vi "Update Joints.vi"(8 "error in (no error)":errorcluster, 9 "Scale (1)":dbl=1.0, 10 "Joints":sgl[](array[numeric]), 11 "Joint Array":T1[](array[typedef])) -> (0 "error out":errorcluster)   [LabVIEW 2017, in "NI_Robotics_3DKinematics.lvlib"]
uses:
  <vilib>/robotics/Kinematics/Plotting/NI_Robotics_3DKinematics.lvlib
  <vilib>/robotics/Kinematics/Plotting/Joint Control.ctl
  <vilib>/robotics/Kinematics/Plotting/Joint Type.ctl
  <vilib>/Analysis/baseanly.llb/Real A x B.vi
  <vilib>/Analysis/_algsub.llb/Vector Norm.vi
  <vilib>/Analysis/_algsub.llb/Real Vector Norm.vi
  <vilib>/Analysis/baseanly.llb/Outer Product.vi
  <vilib>/Analysis/baseanly.llb/Real Outer Product.vi
  <vilib>/robotics/Kinematics/Create Lie Group Matrix.vi
  <vilib>/Utility/AngleManip/Degrees to Radians (Scalar DBL).vi
  <vilib>/Analysis/Matrix/Numeric/Add/Add.vi
  <vilib>/Analysis/Matrix/Numeric/Add/Add - RM,RM.vi
  <vilib>/Analysis/Matrix/Numeric/Multiply/Multiply.vi
  <vilib>/Analysis/Matrix/Numeric/Multiply/Multiply - R,RM.vi
  <vilib>/Analysis/Matrix/Numeric/Multiply/Multiply - RM,R.vi
  <vilib>/Analysis/7linalg.llb/Create Special Matrix.vi
  <vilib>/Analysis/7linalg.llb/Create Special Real Matrix.vi
  <vilib>/picture/3D Picture Control/NI_3D Picture Control.lvlib
  <vilib>/Utility/AngleManip/NI_AngleManipulation.lvlib
  <vilib>/robotics/Kinematics/NI_Kinematics.lvlib
  <vilib>/Analysis/NI_AALBase.lvlib
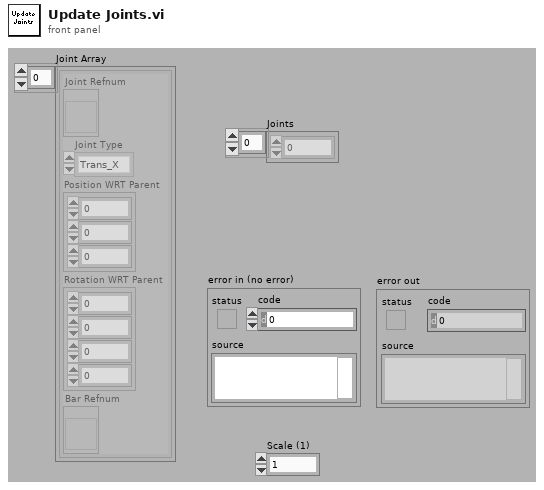
[diagram p1: front panel]
types:
  T1 = typedef "NI_Robotics_3DKinematics.lvlib/Joint Control.ctl" = cluster{"Joint Refnum":refnum<vi>, "Joint Type":T2, "Position WRT Parent":dbl[], "Rotation WRT Parent":dbl[], "Bar Refnum":refnum<vi>}
  T2 = typedef "NI_Robotics_3DKinematics.lvlib/Joint Type.ctl" = enum16{"Trans_X", "Trans_Y", "Trans_Z", "Rot_X", "Rot_Y", "Rot_Z", "None"}
  T3 = cluster{"Position WRT Parent[0]":dbl, "Position WRT Parent[1]":dbl, "Position WRT Parent[2]":dbl}
  T4 = cluster{"Rotation WRT Parent[0]":dbl, "Rotation WRT Parent[1]":dbl, "Rotation WRT Parent[2]":dbl}
  T5 = typedef "NI_Matrix.lvlib/RealMatrix.ctl" = dbl[][]
  T6 = cluster{"A x B[0]":dbl, "A x B[1]":dbl, "A x B[2]":dbl}
  T7 = cluster{"Numeric":dbl, "Numeric":dbl, "Numeric":dbl}
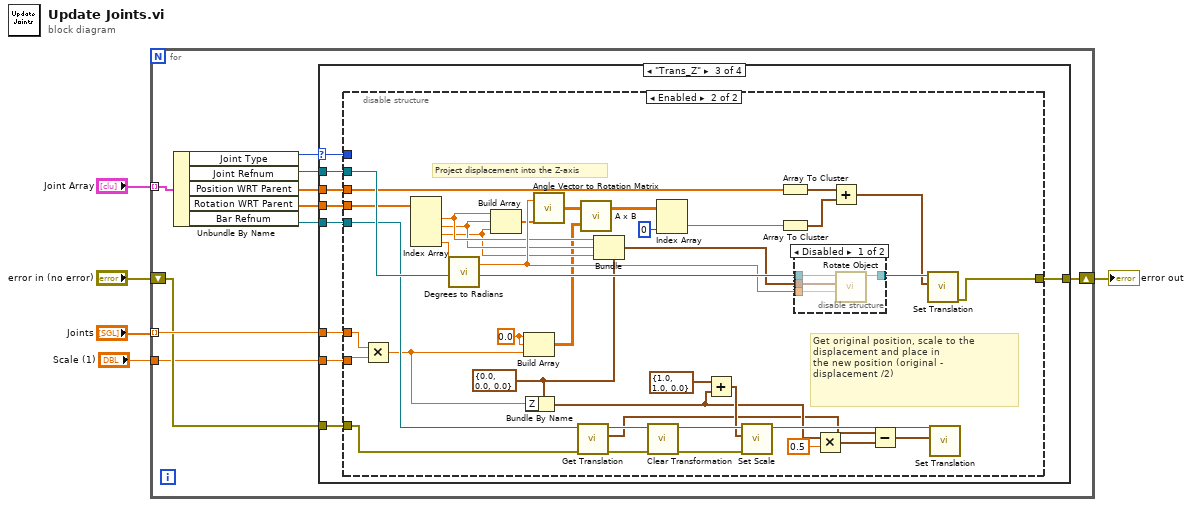
[diagram p0: block diagram]
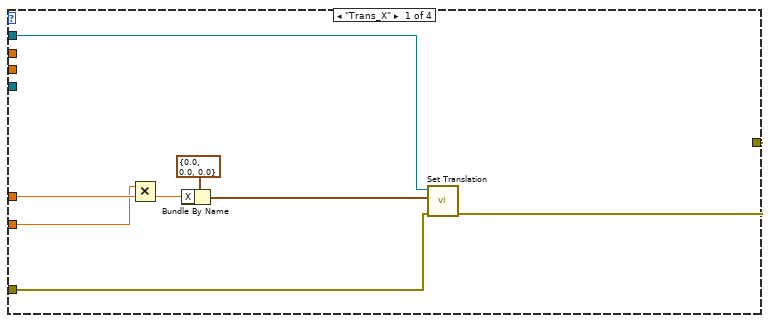
[diagram p2: hidden frame]
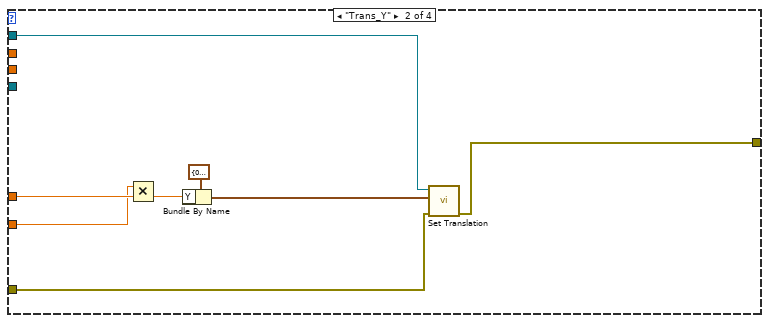
[diagram p3: hidden frame]
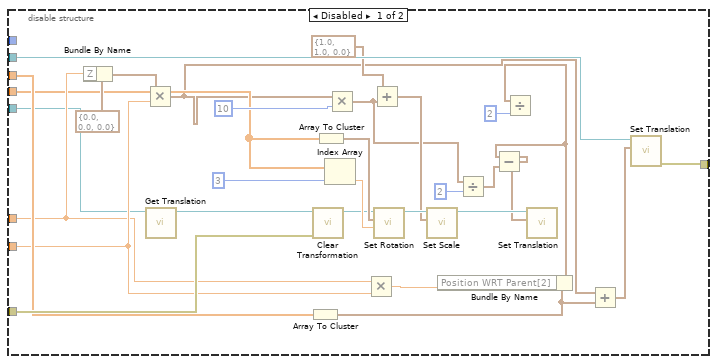
[diagram p4: hidden frame]
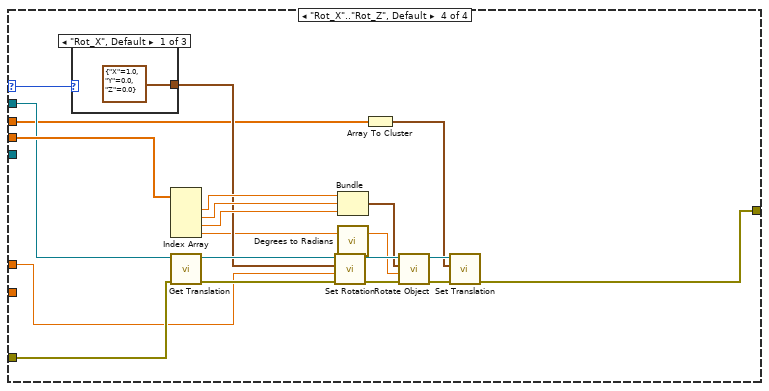
[diagram p6: hidden frame]
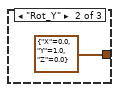
[diagram p7: hidden frame]
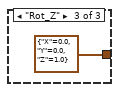
[diagram p8: hidden frame]
diagram:
  n1 = for {
    tunnel: "Joint Array" -> [w14] mode=indexing
    tunnel: "Joints" -> [w15] mode=indexing
    shift-right: [w11] -> w2
    shift-left: "error in (no error)" -> [w8]
    tunnel: "Scale (1)" -> [w6]
    n2 = Unbundle By Name(w14) -> ("Joint Type"=w9:T2, "Joint Refnum"=w10:refnum<vi>, "Position WRT Parent"=w12:dbl[], "Rotation WRT Parent"=w13:dbl[], "Bar Refnum"=w7:refnum<vi>)
    n3 = case shown="\"Trans_Z\"" w9 {
      selector: w9 -> [_ _ w32 w123]
      tunnel: w15 -> [w21 w31 w35 w119]
      tunnel: [w22 w29 w39 w127] -> w11
      tunnel: w13 -> [_ _ w33 w135]
      tunnel: w12 -> [_ _ w37 w115]
      tunnel: w10 -> [w19 w27 w40 w124]
      tunnel: w8 -> [w18 w26 w38 w120]
      tunnel: w7 -> [_ _ w34 _]
      tunnel: w6 -> [w16 w24 w36 _]
      frame "Trans_X" {
        n4 = Multiply(x=w16, y=w21) -> (x*y=w17:dbl)
        n5 = Bundle By Name(cluster=cluster{"X":sgl, "Y":sgl, "Z":sgl} {"X"=0.0, "Y"=0.0, "Z"=0.0} ("Translation"), "X"=w17) -> (w23:cluster{"X":sgl, "Y":sgl, "Z":sgl})
        n6 = call <vilib>:"Set Translation.vi"("error in (no error)"=w18, "Translation"=w23, "Scene Object"=w19) -> ("error out"=w22:errorcluster)  [unwired: 8 out]
      }
      frame "Trans_Y" {
        n7 = Multiply(x=w24, y=w31) -> (x*y=w25:dbl)
        n8 = Bundle By Name(cluster=cluster{"X":sgl, "Y":sgl, "Z":sgl} {"X"=0.0, "Y"=0.0, "Z"=0.0} ("Translation"), "Y"=w25) -> (w30:cluster{"X":sgl, "Y":sgl, "Z":sgl})
        n9 = call <vilib>:"Set Translation.vi"("error in (no error)"=w26, "Translation"=w30, "Scene Object"=w27) -> ("error out"=w29:errorcluster)  [unwired: 8 out]
      }
      frame "Trans_Z" {
        n10 = disable-structure shown="Enabled" {
          disable-tunnel: w40 -> [w69 w106]
          disable-tunnel: [w68 w77] -> w39
          disable-tunnel: w38 -> [w67 w73]
          disable-tunnel: w37 -> [w63 w98]
          disable-tunnel: w36 -> [w60 w108]
          disable-tunnel: w35 -> [w59 w109]
          disable-tunnel: w34 -> [w56 w103]
          disable-tunnel: w33 -> [w54 w102]
          disable-tunnel: w32 -> [_ _]
          frame Disabled {
            n11 = Bundle By Name(cluster=cluster{"X":sgl, "Y":sgl, "Z":sgl} {"X"=0.0, "Y"=0.0, "Z"=0.0} ("Translation"), "Z"=w59) -> (w61:cluster{"X":sgl, "Y":sgl, "Z":sgl})
            n12 = Multiply(x=w61, y=w60) -> (x*y=w42:cluster{"X":dbl, "Y":dbl, "Z":dbl})
            n13 = call <vilib>:"Get Translation.vi"("Scene Object"=w56) -> ("Scene Object"=w55:refnum<vi>)  [unwired: 8 in, 2 out]
            n14 = Array To Cluster(array=w63) -> (cluster=w43:T3)
            n15 = call <vilib>:"Clear Transformation.vi"("error in (no error)"=w67, "Object Refnum In"=w55) -> ("Object Refnum Out"=w50:refnum<vi>)  [unwired: 8 in, 1 out]
            n16 = Array To Cluster(array=w54) -> (cluster=w66:T4)
            n17 = Index Array(array=w54, index=3) -> (element=w64:dbl)
            n18 = Multiply(x=w42, y=10) -> (x*y=w45:cluster{"X":dbl, "Y":dbl, "Z":dbl})
            n19 = Multiply(x=w59, y=w60) -> (x*y=w51:dbl)
            n20 = Add(x=cluster{"X":sgl, "Y":sgl, "Z":sgl} {"X"=1.0, "Y"=1.0, "Z"=0.0} ("Translation"), y=w45) -> (x+y=w46:cluster{"X":dbl, "Y":dbl, "Z":dbl})
            n21 = call <vilib>:"Set Rotation.vi"("Angle"=w64, "Axis"=w66, "Scene Object"=w50) -> ("Rotated Scene Object"=w70:refnum<vi>)  [unwired: 7 in, 1 out]
            n22 = call <vilib>:"Set Scale.vi"("Scale"=w46, "Scene Object"=w70) -> ("Scaled Object"=w49:refnum<vi>)  [unwired: 8 in, 1 out]
            n23 = Bundle By Name(cluster=w43, "Position WRT Parent[2]"=w51) -> (w48:T3)
            n24 = Divide(x=w45, y=2) -> (x/y=w47:cluster{"X":dbl, "Y":dbl, "Z":dbl})
            n25 = Subtract(x=w48, y=w47) -> (x-y=w44:cluster{dbl, dbl, dbl})
            n26 = Divide(x=w48, y=2) -> ()  [unwired: 1 out]
            n27 = call <vilib>:"Set Translation.vi"("Translation"=w44, "Scene Object"=w49) -> ()  [unwired: 8 in, 2 out]
            n28 = Add(x=w42, y=w43) -> (x+y=w41:cluster{dbl, dbl, dbl})
            n29 = call <vilib>:"Set Translation.vi"("Translation"=w41, "Scene Object"=w69) -> ("error out"=w68:errorcluster)  [unwired: 1 in, 8 out]
          }
          frame Enabled {
            w90 = 0.0 ("element")
            w96 = cluster{"X":sgl, "Y":sgl, "Z":sgl} {"X"=0.0, "Y"=0.0, "Z"=0.0} ("Translation")
            # "Get original position, scale to the displacement and place in\nthe new position (original - displacement /2)"
            # "Project displacement into the Z-axis"
            n30 = Multiply(x=w109, y=w108) -> (x*y=w82:dbl)
            n31 = Index Array(array=w102) -> (element #1=w94:dbl, element #2=w93:dbl, element #3=w92:dbl, element #4=w107:dbl)  [unwired: 4 in]
            n32 = call-poly <vilib>:"Degrees to Radians.vi"("angle (deg)"=w107) -> ("angle (rad)"=w95:dbl)  [unwired: 2 in]
            n33 = Build Array(w94, w93, w92) -> (w91:dbl[])
            n34 = Build Array(w90, w90, w82) -> (w88:T5)
            n35 = Bundle By Name(cluster=w96, "Z"=w82) -> (w80:cluster{"X":sgl, "Y":sgl, "Z":sgl})
            n36 = call <vilib>:"Angle Vector to Rotation Matrix.vi"("vector"=w91, "angle"=w95) -> ("rotation matrix"=w89:T5)
            n37 = call <vilib>:"Get Translation.vi"("error in (no error)"=w73, "Scene Object"=w103) -> ("error out"=w72:errorcluster, "Transformation:Get Translation"=w76:cluster{"X":sgl, "Y":sgl, "Z":sgl}, "Scene Object"=w78:refnum<vi>)  [unwired: 7 in]
            n38 = call-poly <vilib>:"A x B.vi"("B"=w88, "A"=w89) -> ("A x B"=w87:T5)  [unwired: 1 out]
            n39 = Bundle(cluster=w96, "X"=w94, "Y"=w93, "Z"=w92) -> (w104:cluster{"X":sgl, "Y":sgl, "Z":sgl})
            n40 = call <vilib>:"Clear Transformation.vi"("error in (no error)"=w72, "Object Refnum In"=w78) -> ("error out"=w71:errorcluster, "Object Refnum Out"=w101:refnum<vi>)  [unwired: 8 in]
            n41 = Index Array(array=w87, index (col)=0 ("disabled index (col)")) -> (element=w85:dbl[])  [unwired: 1 in]
            n42 = Add(x=cluster{"X":sgl, "Y":sgl, "Z":sgl} {"X"=1.0, "Y"=1.0, "Z"=0.0} ("Translation"), y=w80) -> (x+y=w99:cluster{"X":sgl, "Y":sgl, "Z":sgl})
            n43 = call <vilib>:"Set Scale.vi"("error in (no error)"=w71, "Scale"=w99, "Scene Object"=w101) -> ("Scaled Object"=w97:refnum<vi>)  [unwired: 7 in, 1 out]
            n44 = Array To Cluster(array=w98) -> (cluster=w83:T3)
            n45 = Array To Cluster(array=w85) -> (cluster=w81:T6)
            n46 = disable-structure shown="Disabled" {
              disable-tunnel: w104 -> [w113 _]
              disable-tunnel: w95 -> [w112 _]
              disable-tunnel: w106 -> [w111 w114]
              disable-tunnel: [w110 w114] -> w105
              frame Disabled {
                n47 = call <vilib>:"Rotate Object.vi"("Angle"=w112, "Axis"=w113, "Scene.Object In"=w111) -> ("Scene.Object Out"=w110:refnum<vi>)  [unwired: 7 in, 1 out]
              }
              frame Enabled {
              }
            }
            n48 = Multiply(x=w80, y=sgl 0.5 ("cos(x)")) -> (x*y=w74:cluster{"X":sgl, "Y":sgl, "Z":sgl})
            n49 = Add(x=w83, y=w81) -> (x+y=w84:cluster{dbl, dbl, dbl})
            n50 = Subtract(x=w76, y=w74) -> (x-y=w75:cluster{"X":sgl, "Y":sgl, "Z":sgl})
            n51 = call <vilib>:"Set Translation.vi"("Translation"=w84, "Scene Object"=w105) -> ("error out"=w77:errorcluster)  [unwired: 8 in, 1 out]
            n52 = call <vilib>:"Set Translation.vi"("Translation"=w75, "Scene Object"=w97) -> ()  [unwired: 8 in, 2 out]
          }
        }
      }
      frame "Rot_X".."Rot_Z", Default {
        n53 = case shown="\"Rot_X\", Default" w123 {
          tunnel: [cluster{"X":sgl, "Y":sgl, "Z":sgl} {"X"=1.0, "Y"=0.0, "Z"=0.0} ("Axis") cluster{"X":sgl, "Y":sgl, "Z":sgl} {"X"=0.0, "Y"=1.0, "Z"=0.0} ("Axis") cluster{"X":sgl, "Y":sgl, "Z":sgl} {"X"=0.0, "Y"=0.0, "Z"=1.0} ("Axis")] -> w122
          frame "Rot_X", Default {
          }
          frame "Rot_Y" {
          }
          frame "Rot_Z" {
          }
        }
        n54 = Index Array(array=w135) -> (element #1=w132:dbl, element #2=w131:dbl, element #3=w130:dbl, element #4=w117:dbl)  [unwired: 4 in]
        n55 = call <vilib>:"Get Translation.vi"("error in (no error)"=w120, "Scene Object"=w124) -> ("error out"=w128:errorcluster, "Scene Object"=w129:refnum<vi>)  [unwired: 7 in, 1 out]
        n56 = call <vilib>:"Set Rotation.vi"("error in (no error)"=w128, "Angle"=w119, "Axis"=w122, "Scene Object"=w129) -> ("error out"=w134:errorcluster, "Rotated Scene Object"=w133:refnum<vi>)  [unwired: 6 out]
        n57 = Bundle("Numeric"=w132, "Numeric"=w131, "Numeric"=w130) -> (w121:T7)  [unwired: 1 in]
        n58 = call-poly <vilib>:"Degrees to Radians.vi"("angle (deg)"=w117) -> ("angle (rad)"=w118:dbl)  [unwired: 2 in]
        n59 = Array To Cluster(array=w115) -> (cluster=w116:T3)
        n60 = call <vilib>:"Rotate Object.vi"("error in (no error)"=w134, "Angle"=w118, "Axis"=w121, "Scene.Object In"=w133) -> ("error out"=w126:errorcluster, "Scene.Object Out"=w125:refnum<vi>)  [unwired: 6 in]
        n61 = call <vilib>:"Set Translation.vi"("error in (no error)"=w126, "Translation"=w116, "Scene Object"=w125) -> ("error out"=w127:errorcluster)  [unwired: 7 in, 1 out]
      }
    }
  }
  "error out" <- w2
